vi "Message Throughput.vi"() -> ()   [LabVIEW 2019]
uses:
  <vilib>/Skyline/Configuration/Configuration AMQP_class/Open Configuration AMQP.vi
  <vilib>/Skyline/Message/AMQP/sync/Open (Sync).vi
  <vilib>/Skyline/Message/AMQP/NI Skyline Message AMQP (Sync).lvclass
  <vilib>/Skyline/Configuration/Configuration_class/NI Skyline Configuration.lvclass
  <vilib>/Skyline/Message/NI Skyline Message.lvclass
  <vilib>/Skyline/Configuration/Configuration AMQP_class/NI Skyline Configuration AMQP.lvclass
panel:
  in  "Data Array Size":i32=100000
  out "Message Size (Bytes)":i32
  out "Throughput (B/S)":dbl format="%#.2p"
  out "Total Time (Seconds)":dbl
  out "Total Bytes Sent":dbl format="%.2p"
  out "Publish Time":u32(graph)
  out "Messages Published":u32
  in  "Stop":bool
  in  "Test Duration (Seconds)":dbl=30.0
  out "Time to Send File (mS)":u32
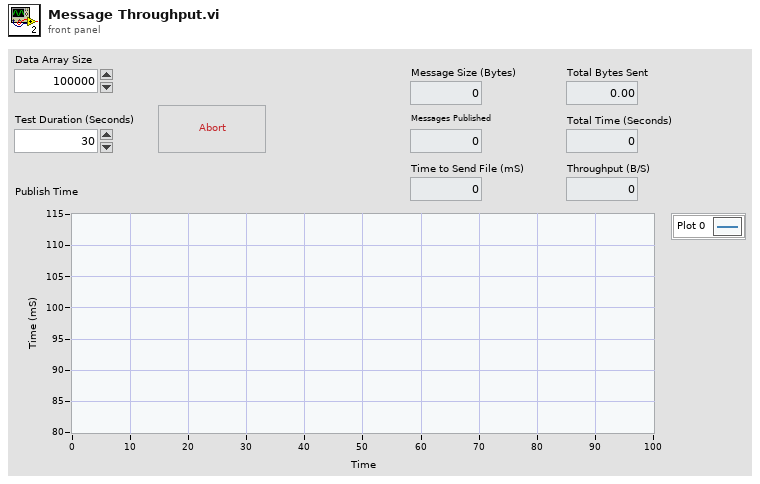
[diagram p1: front panel]
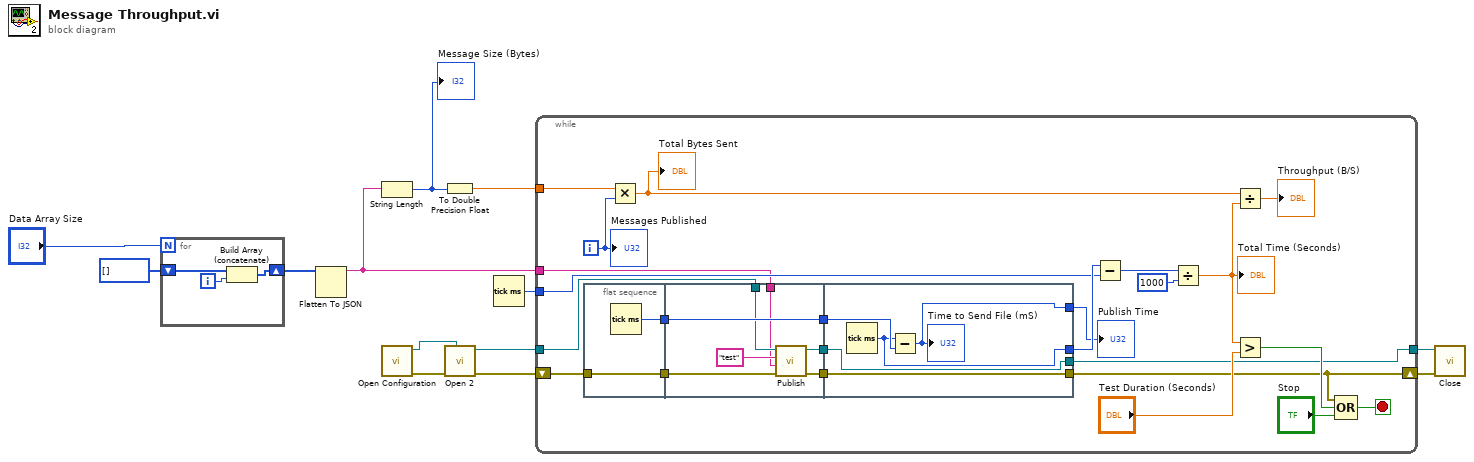
[diagram p0: block diagram]
diagram:
  n1 = for {
    N: "Data Array Size" -> [_]
    shift-right: [w15] -> w11
    shift-left: i32[] [] -> [w14]
    i -> [w16]
    n2 = Build Array (concatenate)(w14, w16) -> (w15:i32[])
  }
  n3 = Flatten To JSON(anything=w11) -> (JSON string=w6:string)  [unwired: 2 in, 1 out]
  n4 = String Length(string=w6) -> (length=w4:i32)
  "Message Size (Bytes)" <- w4
  n5 = call-poly <vilib>:"Open Configuration.vi"() -> ("error out"=w10:errorcluster, "configuration"=w8:refnum<class "NI Skyline Configuration AMQP.lvclass">)  [unwired: 10 in]
  n6 = To Double Precision Float(number=w4) -> (double precision float=w3:dbl)
  n7 = call-poly <vilib>:"Open 2.vi"("configuration"=w8, "error in (no error)"=w10) -> ("error out"=w1:errorcluster, "message session"=w2:refnum<class "NI Skyline Message AMQP (Sync).lvclass">)  [unwired: 8 in]
  n8 = Tick Count (ms)() -> (millisecond timer value=w13:u32)
  n9 = while {
    tunnel: w13 -> [w37]
    tunnel: w2 -> [w25]
    tunnel: [w22] -> w9
    shift-right: [w19] -> w7
    shift-left: w1 -> [w26]
    tunnel: w6 -> [w21]
    tunnel: w3 -> [w20]
    i -> [w33]
    stop <- w17 stop-if-true
    n10 = flat-sequence {
      tunnel: [w42] -> w40
      tunnel: [w41] -> w27
      tunnel: w26 -> [w41]
      tunnel: w40 -> [w49]
      tunnel: [w49] -> w39
      tunnel: w27 -> [w47]
      tunnel: w25 -> [w48]
      tunnel: [w46] -> w24
      tunnel: [w45] -> w23
      tunnel: w21 -> [w43]
      tunnel: w39 -> [w54]
      tunnel: [w53] -> w34
      tunnel: [w52] -> w38
      tunnel: [w51] -> w19
      tunnel: w24 -> [w51]
      tunnel: w23 -> [w50]
      tunnel: [w50] -> w22
      frame #0 {
        n11 = Tick Count (ms)() -> (millisecond timer value=w42:u32)
      }
      frame #1 {
        n12 = call-dynamic "Publish.vi"("error in (no error)"=w47, "message"=w43, "topic"="test", "message session in"=w48) -> ("error out"=w46:errorcluster, "message session out"=w45:refnum<class "NI Skyline Message AMQP (Sync).lvclass">)  [unwired: 6 in]
      }
      frame #2 {
        n13 = Tick Count (ms)() -> (millisecond timer value=w52:u32)
        n14 = Subtract(x=w52, y=w54) -> (x-y=w53:u32)
        "Time to Send File (mS)" <- w53
      }
    }
    n15 = Multiply(x=w20, y=w33) -> (x*y=w32:dbl)
    "Total Bytes Sent" <- w32
    n16 = Subtract(x=w38, y=w37) -> (x-y=w31:u32)
    n17 = Divide(x=w31, y=u32 1000) -> (x/y=w18:dbl)
    "Total Time (Seconds)" <- w18
    n18 = Divide(x=w32, y=w18) -> (x/y=→"Throughput (B/S)":dbl)
    n19 = Greater?(x=w18, y="Test Duration (Seconds)") -> (0:w36:bool)
    n20 = Compound Arithmetic op=OR(w19, w36, "Stop") -> (w17:bool)
    "Messages Published" <- w33
    "Publish Time" <- w34
  }
  n21 = call-dynamic "Close.vi"("error in (no error)"=w7, "message session"=w9) -> ()  [unwired: 9 in, 1 out]
